vi "Update Modbus.vi"(8 "error in":errorcluster, 11 "Modbus":dbl[](array[numeric])) -> (0 "error out":errorcluster)   [LabVIEW 2018, in "UDP Writer.lvlib"]
doc: "This subVI enqueues the named action in to the communications queue along with the input data."
uses:
  UDP Writer.lvlib
  Private Controls/Module Data.ctl
  Private Controls/Module Action.ctl
  f2a7a6e6-2a9f-4252-8788-acfb1c615a21.vi
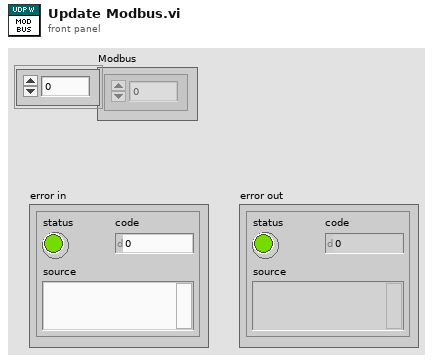
[diagram p1: front panel]
types:
  T1 = typedef "UDP Writer.lvlib/Module Data.ctl" = cluster{"Data":variant, "Action":T2}
  T2 = typedef "UDP Writer.lvlib/Module Action.ctl" = enum16{"Init", "Update ARINC", "Update Waterfall", "Update RPMs", "Update Temps", "Update Modbus", "Update AI", "Update Vibs", "Write", "Error"}
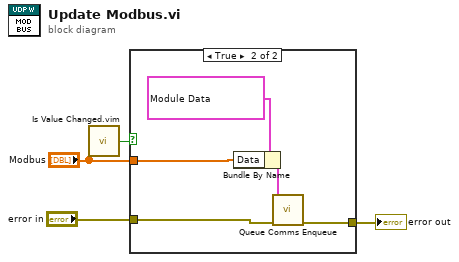
[diagram p0: block diagram]
diagram:
  n1 = call "Is Value Changed.vim"("value"="Modbus") -> ("changed or first call?"=w1:bool)
  n2 = case shown="True" w1 {
    tunnel: [w5 w10] -> w4
    tunnel: "error in" -> [w5 w9]
    tunnel: "Modbus" -> [_ w6]
    frame False {
    }
    frame True {
      n3 = Bundle By Name(cluster=T1 {"Data"=variant, "Action"=enum."Update Modbus"} ("element"), "Data"=w6) -> (w7:T1)
      n4 = call "Queue Comms Enqueue.vi"("error in (no error)"=w9, "element"=w7) -> ("error out"=w10:errorcluster)  [unwired: 9 in]
    }
  }
  "error out" <- w4
